vi "LinearSystemLoop_Pack_Ctrl_Params.vi"(8 "Max Control Effort":dbl[](array[numeric]), 9 "Control Tol":dbl[](array[numeric]), 10 "Measure Std Dev":dbl[](array[numeric]), 11 "Model Std Dev":dbl[](array[numeric])) -> (3 "LinearSystemLoop_Control_Params":T1)   [LabVIEW 2019, in "Trajectory_Library.lvlib"]
doc: "Pack control parameters needed for the Linear System Loop Execute function.\n\nInputs:\n - Model Std Dev -- double array (states) -- Array of standard deviations for model states.\n - Measure Std Dev -- double array(outputs) -- Array of standard devations for model outputs\n - Control Tol -- double array(states) -- Array of standard deviations for controlled model states.\n - Max Control Effort -- double array(inputs) -- Array of maximum values for inputs (classical control outputs) \n\nOutputs:\n - LinearSystemLoopControlParams -- cluster -- Packed values."
uses:
  Trajectory_Library.lvlib
  TypeDef/LINEAR_SYSTEM_LOOP_CTRL_PARAMS.CTL
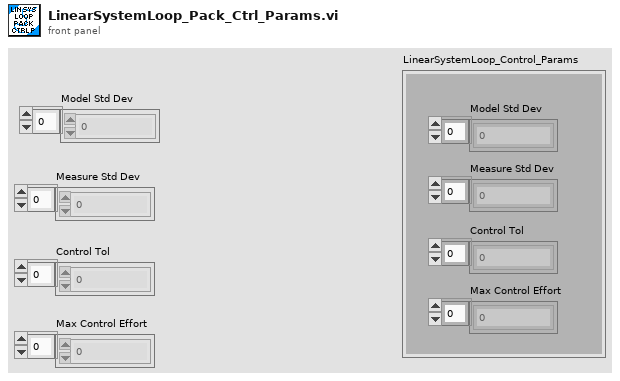
[diagram p1: front panel]
types:
  T1 = typedef "Trajectory_Library.lvlib/LINEAR_SYSTEM_LOOP_CTRL_PARAMS.CTL" = cluster{"Model Std Dev":dbl[], "Measure Std Dev":dbl[], "Control Tol":dbl[], "Max Control Effort":dbl[]}
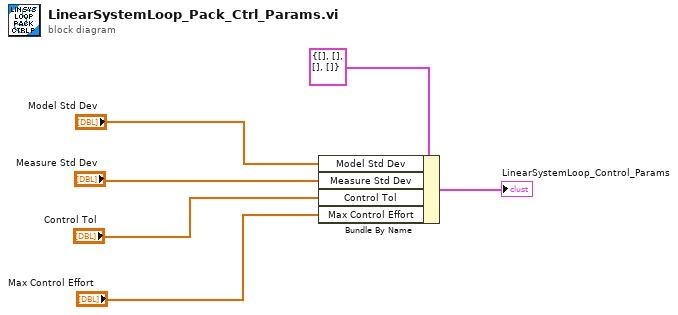
[diagram p0: block diagram]
diagram:
  n1 = Bundle By Name(cluster=T1 {"Model Std Dev"=[], "Measure Std Dev"=[], "Control Tol"=[], "Max Control Effort"=[]} ("LinearSystemLoop_Control_Params"), "Model Std Dev"="Model Std Dev", "Measure Std Dev"="Measure Std Dev", "Control Tol"="Control Tol", "Max Control Effort"="Max Control Effort") -> (→"LinearSystemLoop_Control_Params":T1)
